vi "Test.vi"() -> ()   [LabVIEW 2014]
uses:
  <vilib>/Platform/TimedLoop/XDataNode/timing_clust.ctl
  <vilib>/Platform/TimedLoop/XDataNode/nitl_modes.ctl
  <vilib>/Platform/TimedLoop/XDataNode/wakeup.ctl
  <vilib>/addons/control/pid/pid.llb/PID Advanced (DBL).vi
  <vilib>/platform/TimedLoop/XDataNode/XDataNode.xnode
  <vilib>/addons/control/pid/NI_PID_pid.lvlib
  <vilib>/Platform/TimedLoop/XDataNode/XDNodeRunTimeDep.lvlib
panel:
  out "Sensor Voltage":sgl
  out "Duty Cycle":u32
  in  "Setpoint (V)":dbl
  in  "stop sensor":bool
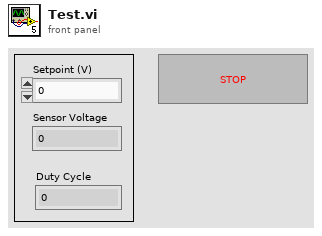
[diagram p1: front panel]
types:
  T1 = typedef "XDNodeRunTimeDep.lvlib/timing_clust.ctl" = cluster{"Expected End [f-1]":u64, "Actual End [f-1]":u64, "Finished Late? [f-1]":bool, "Expected End [i-1]":u64, "Actual End [i-1]":u64, "Finished Late? [i-1]":bool, "Expected Start [i]":u64, "Actual Start [i]":u64, "Expected Start [f]":u64, "Actual Start [f]":u64, "Source Name":string, "Structure Name":string, "Period":i64, "Deadline":i64, "Offset":i64, "Start":i64, "Priority":i32, "Timeout":i32, "Mode":T2, "Wakeup Reason":T3, "Error":errorcluster, "Source Type":string, "Secondary Source Type":string, "Global End Time":u64, "Global Start Time":u64, "Frame Duration":u64, "Iteration Duration":u64, "Assigned CPU":i32, "I/O Scan Engine Mode":u32}
  T2 = typedef "XDNodeRunTimeDep.lvlib/nitl_modes.ctl" = enum32{"No Change", "Process missed periods, maintain original phase", "Discard missed periods, maintain original phase", "Process missed periods, ignore original phase", "Discard missed periods, ignore original phase"}
  T3 = typedef "XDNodeRunTimeDep.lvlib/wakeup.ctl" = enum32{"Normal", "Aborted", "Asynchronous wakeup", "Timing source error", "Timed loop error", "Timeout"}
  T4 = cluster{"proportional gain (Kc)":dbl, "integral time (Ti, min)":dbl, "derivative time (Td, min)":dbl}
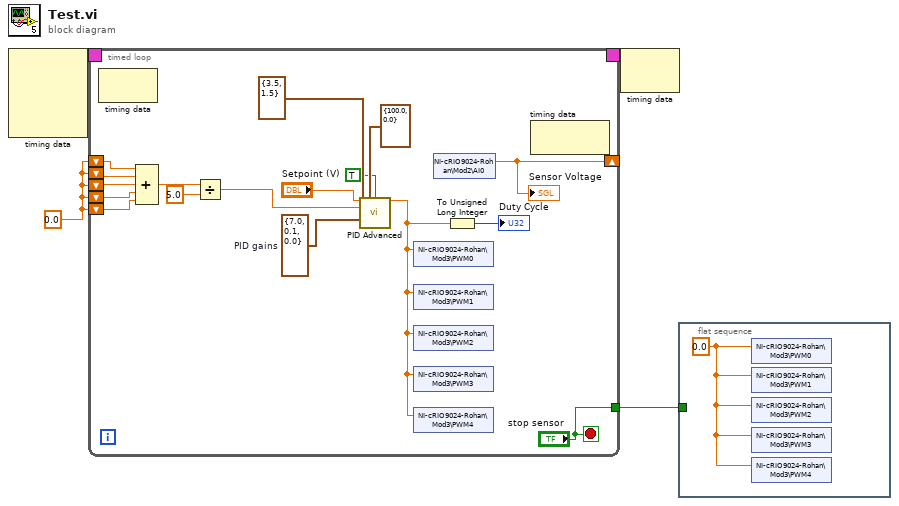
[diagram p0: block diagram]
diagram:
  w4 = 0.0
  n1 = node-c288() -> (w2:T1)  [unwired: 4 in]
  n2 = timed-loop {
    shift-right: [w5] -> _
    shift-left: w4 -> [w21]
    shift-left: w4 -> [w20]
    shift-left: w4 -> [w19]
    shift-left: w4 -> [w18]
    shift-left: w4 -> [w17]
    tunnel: ["stop sensor"] -> w3
    timing: w2 -> [_]
    timing-out: [_] -> w1
    stop <- "stop sensor" stop-if-true
    w14 = T4 {"proportional gain (Kc)"=7.0, "integral time (Ti, min)"=0.1, "derivative time (Td, min)"=0.0}  # PID gains
    n3 = node-c288() -> ()  [unwired: 1 in, 1 out]
    n4 = Compound Arithmetic op=ADD(w21, w20, w19, w18, w17) -> (w16:dbl)
    n5 = Divide(x=w16, y=5.0) -> (x/y=w12:dbl)
    n6 = call-poly <vilib>:"PID Advanced.vi"("setpoint"="Setpoint (V)", "output range"=cluster{"output high":dbl, "output low":dbl} {"output high"=100.0, "output low"=0.0}, "auto? (T)"=TRUE, "process variable"=w12, "setpoint range"=cluster{"setpoint high":dbl, "setpoint low":dbl} {"setpoint high"=3.5, "setpoint low"=1.5}, "PID gains"=w14) -> ("output"=w8:dbl)  [unwired: 8 in, 1 out]
    n7 = shared-variable "NI-cRIO9024-Rohan\\Mod3\\PWM0"(w8) -> ()  [unwired: 1 in, 1 out]
    n8 = shared-variable "NI-cRIO9024-Rohan\\Mod3\\PWM1"(w8) -> ()  [unwired: 1 in, 1 out]
    n9 = shared-variable "NI-cRIO9024-Rohan\\Mod3\\PWM2"(w8) -> ()  [unwired: 1 in, 1 out]
    n10 = shared-variable "NI-cRIO9024-Rohan\\Mod3\\PWM3"(w8) -> ()  [unwired: 1 in, 1 out]
    n11 = shared-variable "NI-cRIO9024-Rohan\\Mod3\\PWM4"(w8) -> ()  [unwired: 1 in, 1 out]
    n12 = shared-variable "NI-cRIO9024-Rohan\\Mod2\\AI0"() -> (w5:dbl)  [unwired: 1 in, 1 out]
    "Sensor Voltage" <- w5
    n13 = To Unsigned Long Integer(number=w8) -> (unsigned 32bit integer=→"Duty Cycle":u32)
    n14 = node-c288() -> ()  [unwired: 1 in, 1 out]
  }
  n15 = node-c288(w1) -> ()  [unwired: 1 out]
  n16 = flat-sequence {
    tunnel: w3 -> [_]
    frame #0 {
      w24 = 0.0 ("PWM0")
      n17 = shared-variable "NI-cRIO9024-Rohan\\Mod3\\PWM0"(w24) -> ()  [unwired: 1 in, 1 out]
      n18 = shared-variable "NI-cRIO9024-Rohan\\Mod3\\PWM1"(w24) -> ()  [unwired: 1 in, 1 out]
      n19 = shared-variable "NI-cRIO9024-Rohan\\Mod3\\PWM2"(w24) -> ()  [unwired: 1 in, 1 out]
      n20 = shared-variable "NI-cRIO9024-Rohan\\Mod3\\PWM3"(w24) -> ()  [unwired: 1 in, 1 out]
      n21 = shared-variable "NI-cRIO9024-Rohan\\Mod3\\PWM4"(w24) -> ()  [unwired: 1 in, 1 out]
    }
  }
